vi "Get 7260 Formated Parameters.VI"(8 "error in (no error)":errorcluster, 10 "Initial String":string, 11 "VISA Resource Name":refnum<visa-resource-name>) -> (0 "error out":errorcluster, 1 "Sensitivity":dbl format="%.4e", 2 "Frequency":dbl format="%.2e", 3 "Parameters":string, 4 "Time Constant":dbl format="%.2e", 5 "Oscillator voltage":dbl format="%.2e", 6 "Data titles":string[](array[string])=["EGG7260_Vx (V)", "EGG7260_Vy (V)"], 7 "VISA Resource Name Out":refnum<visa-resource-name>)   [LabVIEW 2015]
uses:
  GPIB/VISA  Send Receive.vi
panel:
  out "Ref. phase":dbl format="%.2f"
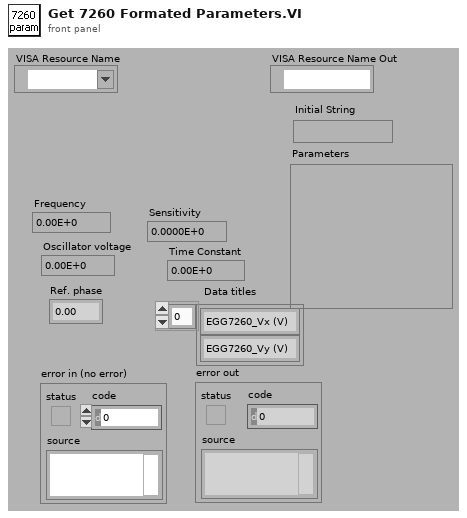
[diagram p1: front panel]
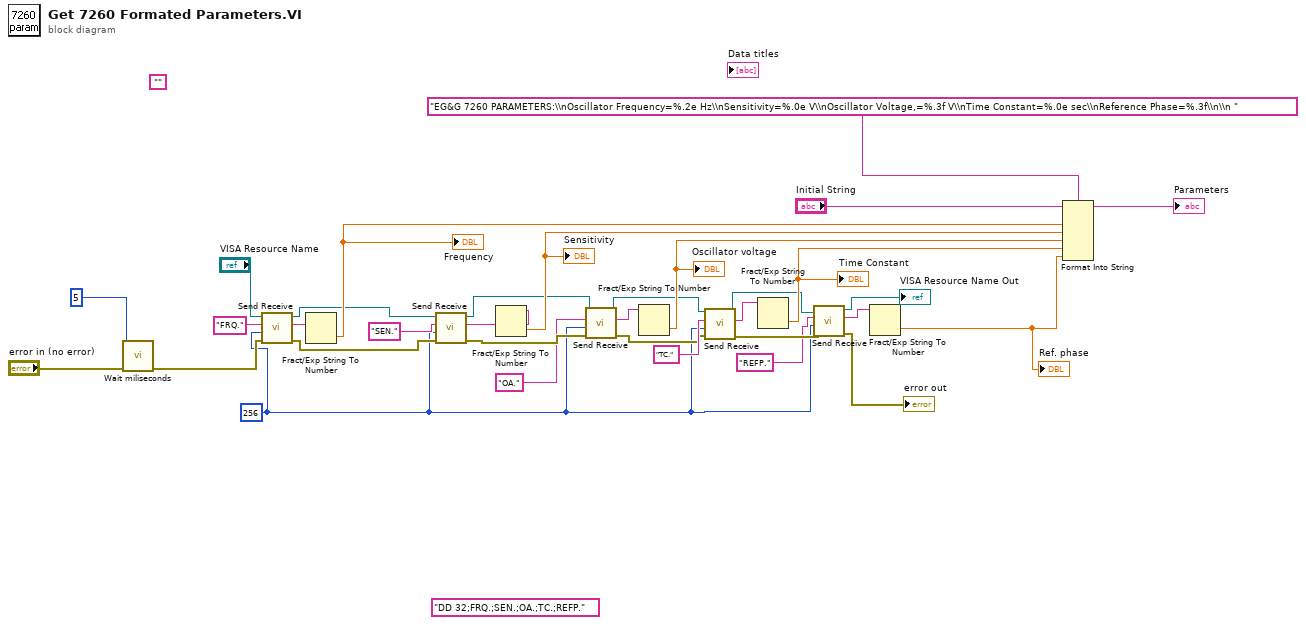
[diagram p0: block diagram]
diagram:
  w4 = 256 ("count")
  (unwired) "DD 32;FRQ.;SEN.;OA.;TC.;REFP." ("data string")
  (unwired) ""
  n1 = call "Wait miliseconds.vi"("error in (no error)"="error in (no error)", "milliseconds to wait"=u32 5) -> ("error out"=w30:errorcluster)  [unwired: 8 in, 1 out]
  n2 = call-poly "Send Receive.vi"("error in (no error)"=w30, "Receive count"=w4, "data string in"="FRQ." ("data string"), "VISA Resource Name"="VISA Resource Name") -> ("error out"=w18:errorcluster, "data string out"=w21:string, "VISA Resource Name Out"=w20:refnum<visa-resource-name>)  [unwired: 5 in]
  n3 = Fract/Exp String To Number(string=w21) -> (number=w27:dbl)  [unwired: 4 out]
  "Frequency" <- w27
  n4 = call-poly "Send Receive.vi"("error in (no error)"=w18, "Receive count"=w4, "data string in"="SEN." ("data string"), "VISA Resource Name"=w20) -> ("error out"=w16:errorcluster, "data string out"=w17:string, "VISA Resource Name Out"=w14:refnum<visa-resource-name>)  [unwired: 5 in]
  n5 = Fract/Exp String To Number(string=w17) -> (number=w26:dbl)  [unwired: 4 out]
  "Sensitivity" <- w26
  n6 = call-poly "Send Receive.vi"("error in (no error)"=w16, "Receive count"=w4, "data string in"="OA." ("data string"), "VISA Resource Name"=w14) -> ("error out"=w11:errorcluster, "data string out"=w13:string, "VISA Resource Name Out"=w10:refnum<visa-resource-name>)  [unwired: 5 in]
  n7 = Fract/Exp String To Number(string=w13) -> (number=w25:dbl)  [unwired: 4 out]
  "Oscillator voltage" <- w25
  n8 = call-poly "Send Receive.vi"("error in (no error)"=w11, "Receive count"=w4, "data string in"="TC." ("data string"), "VISA Resource Name"=w10) -> ("error out"=w8:errorcluster, "data string out"=w9:string, "VISA Resource Name Out"=w7:refnum<visa-resource-name>)  [unwired: 5 in]
  n9 = Fract/Exp String To Number(string=w9) -> (number=w24:dbl)  [unwired: 4 out]
  "Time Constant" <- w24
  n10 = call-poly "Send Receive.vi"("error in (no error)"=w8, "Receive count"=w4, "data string in"="REFP." ("data string"), "VISA Resource Name"=w7) -> ("error out"=→"error out":errorcluster, "data string out"=w5:string, "VISA Resource Name Out"=→"VISA Resource Name Out":refnum<visa-resource-name>)  [unwired: 5 in]
  n11 = Fract/Exp String To Number(string=w5) -> (number=w23:dbl)  [unwired: 4 out]
  "Ref. phase" <- w23
  n12 = Format Into String(format string="EG&G 7260 PARAMETERS:\\nOscillator Frequency=%.2e Hz\\nSensitivity=%.0e V\\nOscillator Voltage,=%.3f V\\nTime Constant=%.0e sec\\nReference Phase=%.3f\\n\\n ", initial string="Initial String", w27, w26, w25, w24, w23) -> (resulting string=→"Parameters":string)  [unwired: 1 in, 1 out]
